vi "Get Forward Offset.vi"(8 "error in (no error)":errorcluster, 11 "caster wheel in":refnum<class "NI_Robotics_Caster Wheel.lvclass">) -> (0 "error out":errorcluster, 2 "forward offset":dbl, 3 "caster wheel out":refnum<class "NI_Robotics_Caster Wheel.lvclass">)   [LabVIEW 2017, in "NI_Robotics_Caster Wheel.lvclass"]
uses:
  <vilib>/robotics/Steering/Caster Wheel/NI_Robotics_Caster Wheel.lvclass
  <vilib>/robotics/Steering/Caster Wheel/NI_Robotics_Caster Wheel.lvclass/NI_Robotics_Caster Wheel.ctl
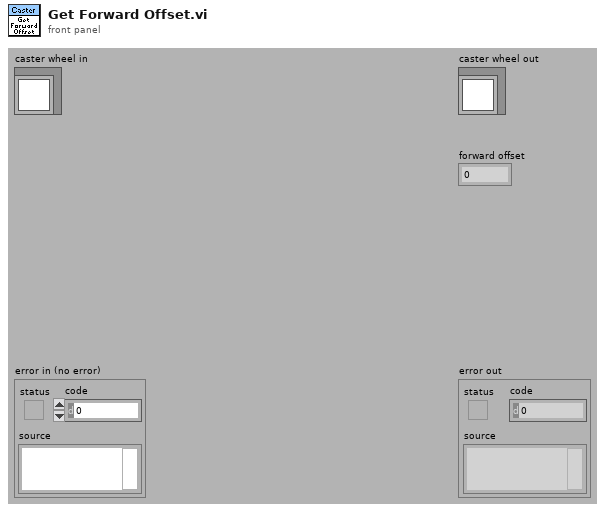
[diagram p1: front panel]
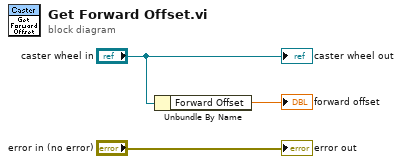
[diagram p0: block diagram]
diagram:
  n1 = Unbundle By Name("caster wheel in") -> ("Forward Offset"=→"forward offset":dbl)
  "error out" <- "error in (no error)"
  "caster wheel out" <- "caster wheel in"
